vi "Tree Add File Infor.vi"(8 "error in (no error)":errorcluster, 11 "[V]System Tree View in":refnum<class "[V]System Tree View.lvclass">) -> (0 "error out":errorcluster, 3 "[V]System Tree View out":refnum<class "[V]System Tree View.lvclass">)   [LabVIEW 2020, in "[V]System Tree View.lvlib" / "[V]System Tree View.lvclass"]
uses:
  [V]System Tree View.lvclass
  Control/Tree Item.ctl
  [V]System Tree View.lvclass/[V]System Tree View.ctl
  Models/Data List/Data List.lvclass/Data List.ctl
  Models/Data List/Accessors/Read Table Name.vi
  Models/Data List/Accessors/Read Channels Names.vi
  Models/Data List/Data List.lvclass
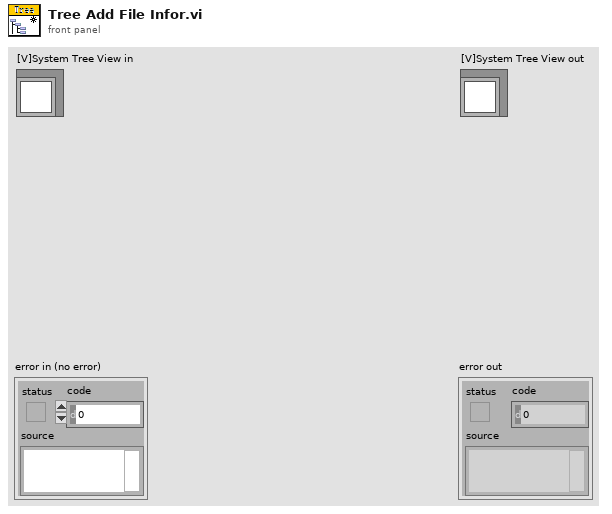
[diagram p1: front panel]
types:
  T1 = typedef "[V]System Tree View.lvlib/[V]System Tree View.lvclass/Tree Item.ctl" = cluster{"Self Tag":string, "Parent Tag":string, "LeftCell Value":string, "RightCells Value":string[], "Is Child":bool, "Symbol Index":i32}
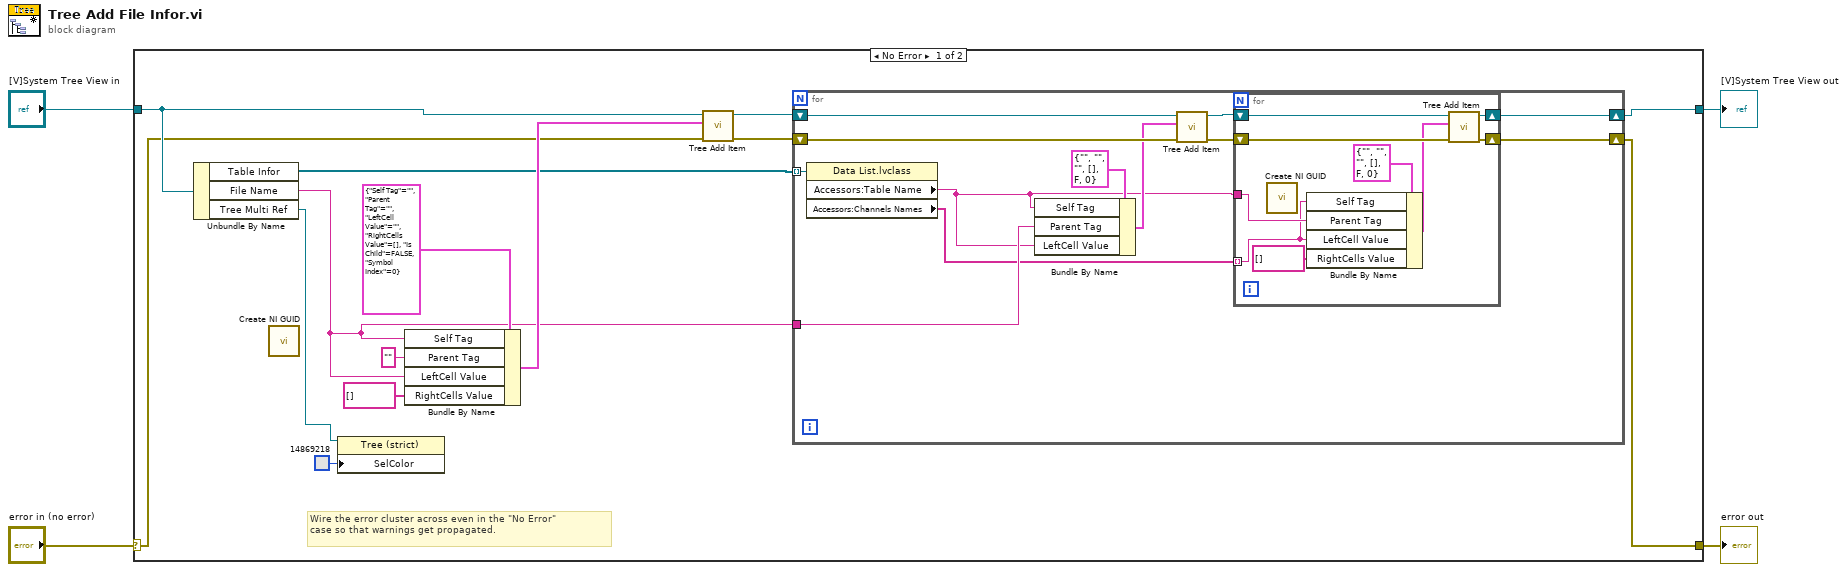
[diagram p0: block diagram]
diagram:
  n1 = case shown="No Error" "error in (no error)" {
    selector: "error in (no error)" -> [w6 w41]
    tunnel: [w11 w41] -> w3
    tunnel: [w12 w40] -> w1
    tunnel: "[V]System Tree View in" -> [w18 w40]
    frame No Error {
      # "Wire the error cluster across even in the \"No Error\"\ncase so that warnings get propagated."
      n2 = Unbundle By Name(w18) -> ("Table Infor"=w7:refnum<class "Data List.lvclass">[], "File Name"=w5:string, "Tree Multi Ref"=w9:refnum<vi>)
      n3 = call <vilib>:"Create NI GUID.vi"() -> ()  [unwired: 1 out]
      n4 = property class="Tree (strict)"(reference=w9, "SelColor"=u32 14869218 ("Selection Color")) -> ()  [unwired: 1 in, 2 out]
      n5 = Bundle By Name(cluster=T1 {"Self Tag"="", "Parent Tag"="", "LeftCell Value"="", "RightCells Value"=[], "Is Child"=FALSE, "Symbol Index"=0} ("Item Map"), "Self Tag"=w5, "Parent Tag"="", "LeftCell Value"=w5, "RightCells Value"=string[] []) -> (w16:T1)
      n6 = call "Tree Add Item.vi"("error in (no error)"=w6, "Item Map"=w16, "[V]System Tree View in"=w18) -> ("error out"=w13:errorcluster, "[V]System Tree View out"=w14:refnum<class "[V]System Tree View.lvclass">)  [unwired: 7 in]
      n7 = for {
        tunnel: w7 -> [w30] mode=indexing
        shift-right: [w21] -> w12
        shift-left: w14 -> [w29]
        shift-right: [w20] -> w11
        shift-left: w13 -> [w28]
        tunnel: w5 -> [w26]
        n8 = property class="Data List.lvclass"(reference=w30) -> ("Accessors:Table Name"=w19:string, "Accessors:Channels Names"=w22:string[])  [unwired: 1 in, 2 out]
        n9 = Bundle By Name(cluster=T1 {"Self Tag"="", "Parent Tag"="", "LeftCell Value"="", "RightCells Value"=[], "Is Child"=FALSE, "Symbol Index"=0} ("Item Map"), "Self Tag"=w19, "Parent Tag"=w26, "LeftCell Value"=w19) -> (w24:T1)
        n10 = call "Tree Add Item.vi"("error in (no error)"=w28, "Item Map"=w24, "[V]System Tree View in"=w29) -> ("error out"=w23:errorcluster, "[V]System Tree View out"=w25:refnum<class "[V]System Tree View.lvclass">)  [unwired: 7 in]
        n11 = for {
          shift-right: [w38] -> w21
          shift-left: w25 -> [w39]
          shift-right: [w36] -> w20
          shift-left: w23 -> [w37]
          tunnel: w19 -> [w34]
          tunnel: w22 -> [w31] mode=indexing
          n12 = call <vilib>:"Create NI GUID.vi"() -> ()  [unwired: 1 out]
          n13 = Bundle By Name(cluster=T1 {"Self Tag"="", "Parent Tag"="", "LeftCell Value"="", "RightCells Value"=[], "Is Child"=FALSE, "Symbol Index"=0} ("Item Map"), "Self Tag"=w31, "Parent Tag"=w34, "LeftCell Value"=w31, "RightCells Value"=string[] []) -> (w33:T1)
          n14 = call "Tree Add Item.vi"("error in (no error)"=w37, "Item Map"=w33, "[V]System Tree View in"=w39) -> ("error out"=w36:errorcluster, "[V]System Tree View out"=w38:refnum<class "[V]System Tree View.lvclass">)  [unwired: 7 in]
        }
      }
    }
    frame Error {
    }
  }
  "error out" <- w3
  "[V]System Tree View out" <- w1
